vi "Self-Test.vi"(8 "error in (no error)":errorcluster, 11 "VISA resource name":refnum<visa-resource-name>) -> (0 "error out":errorcluster, 1 "Self-Test Result Message":string, 2 "Self-Test Result Code":i32, 3 "VISA resource name out":refnum<visa-resource-name>)   [LabVIEW 2013, in "California Instruments iX Series.lvlib"]
doc: "Runs the instrument's self-test routine and returns the test results."
uses:
  California Instruments iX Series.lvlib
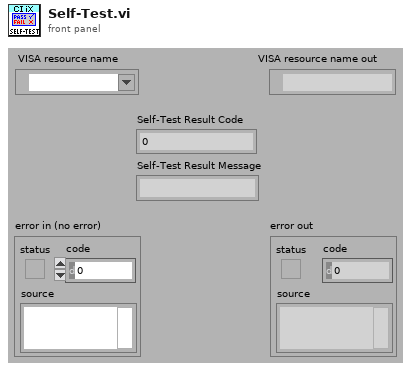
[diagram p1: front panel]
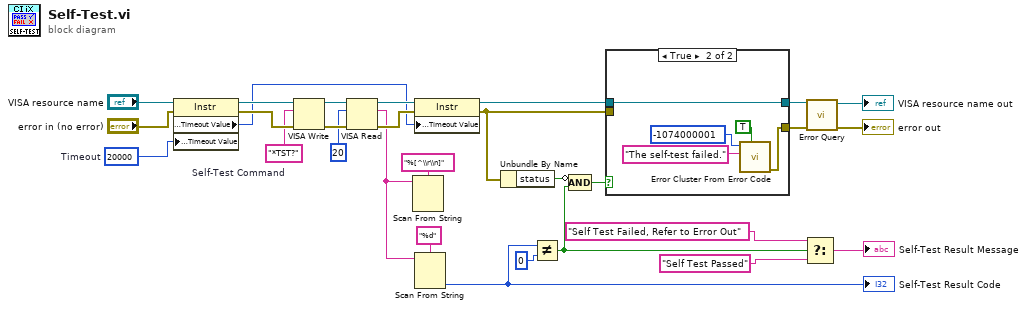
[diagram p0: block diagram]
diagram:
  w17 = u32 20000  # Timeout
  w13 = "*TST?"  # Self-Test Command
  n1 = property class="Instr"(reference="VISA resource name", error in="error in (no error)", "General Settings:Timeout Value"=w17) -> (reference out=w15:refnum<visa-resource-name>, error out=w16:errorcluster, "General Settings:Timeout Value"=w14:u32)
  n2 = VISA Write(VISA resource name=w15, write buffer=w13, error in (no error)=w16) -> (VISA resource name out=w25:refnum<visa-resource-name>, error out=w24:errorcluster)  [unwired: 1 out]
  n3 = VISA Read(VISA resource name=w25, byte count=u32 20 ("byte count (20)"), error in (no error)=w24) -> (VISA resource name out=w27:refnum<visa-resource-name>, read buffer=w20:string, error out=w26:errorcluster)  [unwired: 1 out]
  n4 = Scan From String(format string="%[^\\r\\n]" ("Format String"), input string=w20) -> ()  [unwired: 4 in, 3 out]
  n5 = property class="Instr"(reference=w27, error in=w26, "General Settings:Timeout Value"=w14) -> (reference out=w12:refnum<visa-resource-name>, error out=w11:errorcluster)
  n6 = Scan From String(format string="%d", input string=w20) -> (output 1=w6:i32)  [unwired: 3 in, 3 out]
  "Self-Test Result Code" <- w6
  n7 = Unbundle By Name(w11) -> ("status"=w8:bool)
  n8 = Not Equal?(x=w6, y=0) -> (x != y?=w4:bool)
  n9 = Compound Arithmetic op=AND(invert w8, w4) -> (w7:bool)
  n10 = case shown="True" w7 {
    tunnel: w12 -> [w31 w36]
    tunnel: w11 -> [w30 _]
    tunnel: [w30 w32] -> w10
    tunnel: [w31 w36] -> w9
    frame False {
    }
    frame True {
      n11 = call <vilib>:"Error Cluster From Error Code.vi"("show call chain? (False)"=TRUE, "error message (\"\")"="The self-test failed." ("Source (VI Name)"), "error code (0)"=-1074000001 ("Code")) -> ("error out"=w32:errorcluster)  [unwired: 6 in]
    }
  }
  n12 = Select(t="Self Test Failed, Refer to Error Out", s=w4, f="Self Test Passed") -> (s? t:f=→"Self-Test Result Message":string)
  n13 = call "Error Query.vi"("error in (no error)"=w10, "VISA resource name"=w9) -> ("error out"=→"error out":errorcluster, "VISA resource name out"=→"VISA resource name out":refnum<visa-resource-name>)  [unwired: 6 in, 2 out]
